vi "Merge Graph Data Array.vi"(10 "Graph Data Array":T1[](array[typedef])) -> (1 "Merged Graph Data":T1)   [LabVIEW 2013, in "Diode Characterization.lvlib" / "Diode IV.lvclass"]
doc: "Takes an array of graph data and combines the elements to make one merged graph data output.\n\nThis is useful for combining the output of multiple different analysis routines with the original data."
uses:
  Diode IV.lvclass
  graphdata.ctl
  <vilib>/Utility/miscctls.llb/LVAnnotationListTypeDef.ctl
  <vilib>/Utility/miscctls.llb/LVCursorListTypeDef.ctl
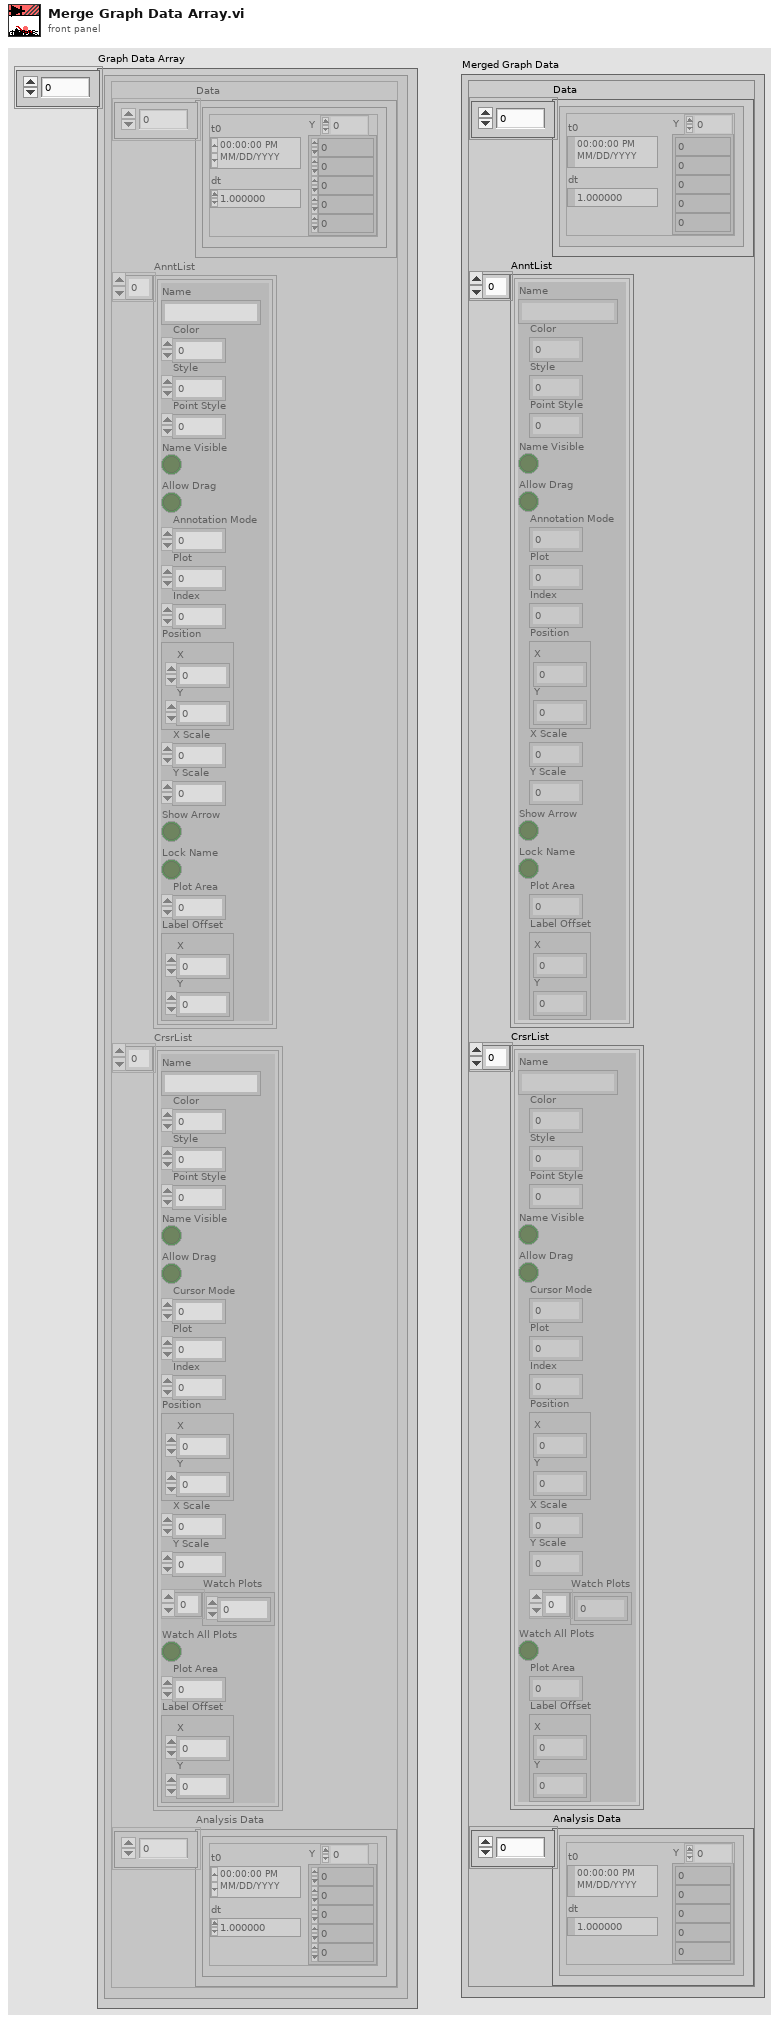
[diagram p1: front panel]
types:
  T1 = typedef "Diode Characterization.lvlib/Diode IV.lvclass/graphdata.ctl" = cluster{"Data":waveform(dbl)[], "AnntList":T2, "CrsrList":T3, "Analysis Data":waveform(dbl)[]}
  T2 = typedef "LVAnnotationListTypeDef.ctl" = cluster{"Name":string, "Color":u32, "Style":u8, "Point Style":u8, "Name Visible":bool, "Allow Drag":bool, "Annotation Mode":u32, "Plot":i32, "Index":i32, "Position":cluster{"X":dbl, "Y":dbl}, "X Scale":u32, "Y Scale":u32, "Show Arrow":bool, "Lock Name":bool, "Plot Area":i32, "Label Offset":cluster{"X":dbl, "Y":dbl}}[]
  T3 = typedef "LVCursorListTypeDef.ctl" = cluster{"Name":string, "Color":u32, "Style":u8, "Point Style":u8, "Name Visible":bool, "Allow Drag":bool, "Cursor Mode":u32, "Plot":i32, "Index":i32, "Position":cluster{"X":dbl, "Y":dbl}, "X Scale":u32, "Y Scale":u32, "Watch Plots":i32[], "Watch All Plots":bool, "Plot Area":i32, "Label Offset":cluster{"X":dbl, "Y":dbl}}[]
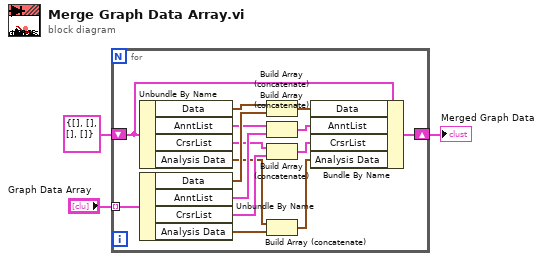
[diagram p0: block diagram]
diagram:
  n1 = for {
    tunnel: "Graph Data Array" -> [w18] mode=indexing
    shift-right: [w16] -> w1
    shift-left: T1 {"Data"=[], "AnntList"=[], "CrsrList"=[], "Analysis Data"=[]} ("Merged Graph Data 2") -> [w17]
    n2 = Unbundle By Name(w17) -> ("Data"=w15:waveform(dbl)[], "AnntList"=w12:T2, "CrsrList"=w9:T3, "Analysis Data"=w6:waveform(dbl)[])
    n3 = Unbundle By Name(w18) -> ("Data"=w13:waveform(dbl)[], "AnntList"=w11:T2, "CrsrList"=w8:T3, "Analysis Data"=w5:waveform(dbl)[])
    n4 = Build Array (concatenate)(w15, w13) -> (w14:waveform(dbl)[])
    n5 = Build Array (concatenate)(w12, w11) -> (w10:T2)
    n6 = Build Array (concatenate)(w9, w8) -> (w7:T3)
    n7 = Build Array (concatenate)(w6, w5) -> (w4:waveform(dbl)[])
    n8 = Bundle By Name(cluster=w17, "Data"=w14, "AnntList"=w10, "CrsrList"=w7, "Analysis Data"=w4) -> (w16:T1)
  }
  "Merged Graph Data" <- w1
